vi "2ASK - 2PSK -2FSK.vi"() -> ()   [LabVIEW 2024]
uses:
  <vilib>/Analysis/NI_AALBase.lvlib
panel:
  in  "Stop":bool
  in  "nbre d'échantillons":i32=1000
  in  "Fréquence (f)":dbl=20.0
  in  "Amplitude (A)":dbl=4.0
  in  "Fréquence (f0)":dbl=20.0
  in  "Fréquence (f1)":dbl=60.0
  in  "nbre d'échantillons":i32=1000
  in  "Amplitude (A)":dbl=5.0
  out "Suite binaire (LED)":bool[](array[boolean]) caption="Array 4"
  in  "Fréquence (f)":dbl=40.0
  in  "nbre d'échantillons":i32=1000
  in  "Amplitude (A0)":dbl=2.0
  in  "Amplitude (A1)":dbl=8.0
  in  "Type de Modulation":u16(ring) items=["2-FSK", "2-PSK", "2-ASK"]
  out "Signal Résultant":dbl[](graph)
  out "Signal Porteur N°1":dbl[](graph)
  out "Inverse du signal binaire x Signal porteur N°2":dbl[](graph)
  out "Signal binaire":dbl[](graph)
  out "Signal Porteur N°2":dbl[](graph)
  out "Signal binaire x Signal porteur N°1":dbl[](graph)
  in  "Suite binaire":bool[](array[boolean])=[TRUE, TRUE, TRUE, FALSE, FALSE, FALSE, FALSE, TRUE, TRUE, TRUE]
  # "Paramètres des signaux porteurs"
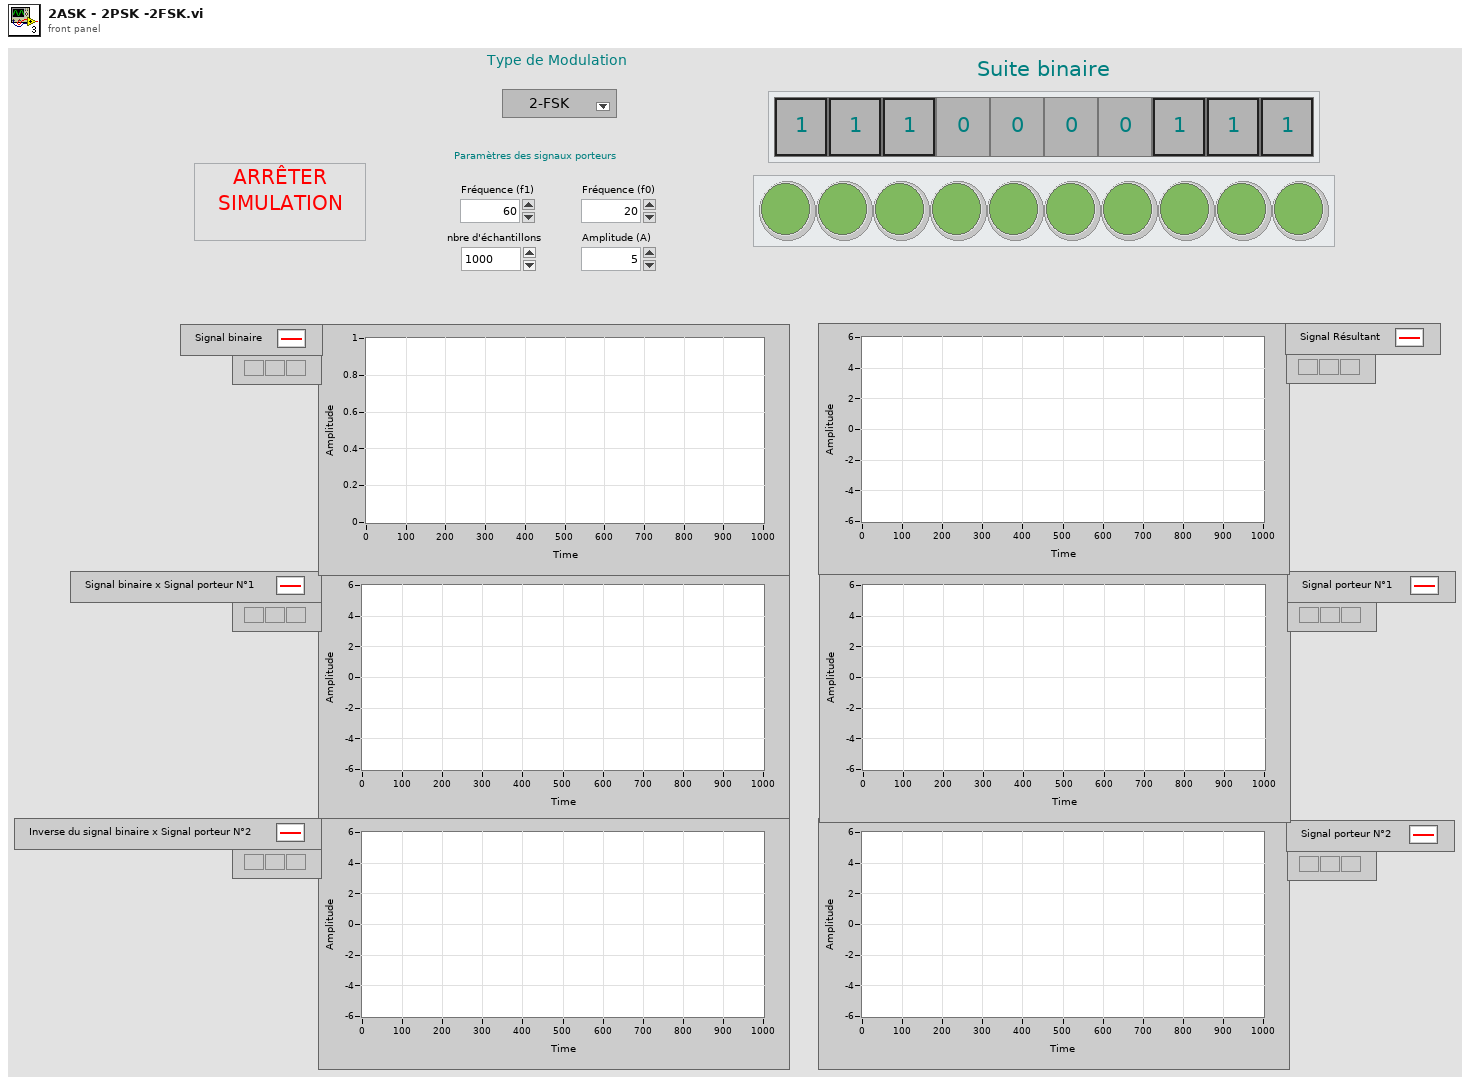
[diagram p1: front panel]
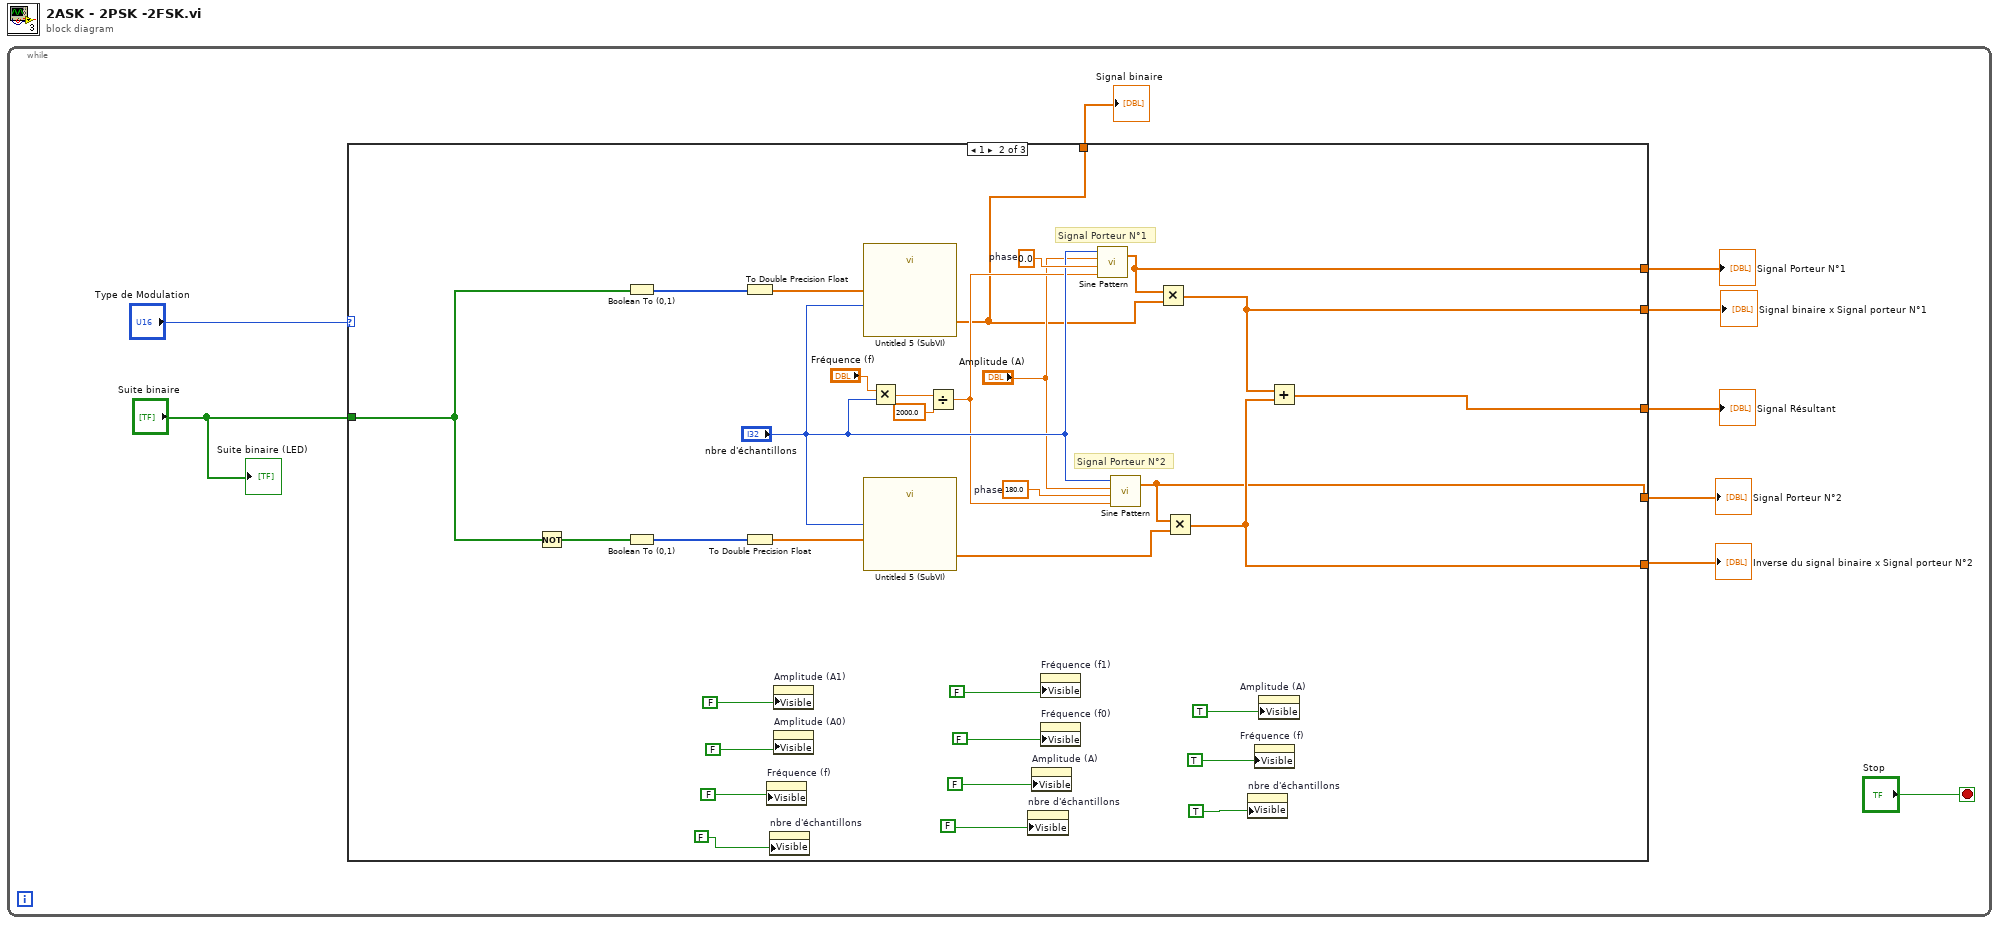
[diagram p0: block diagram]
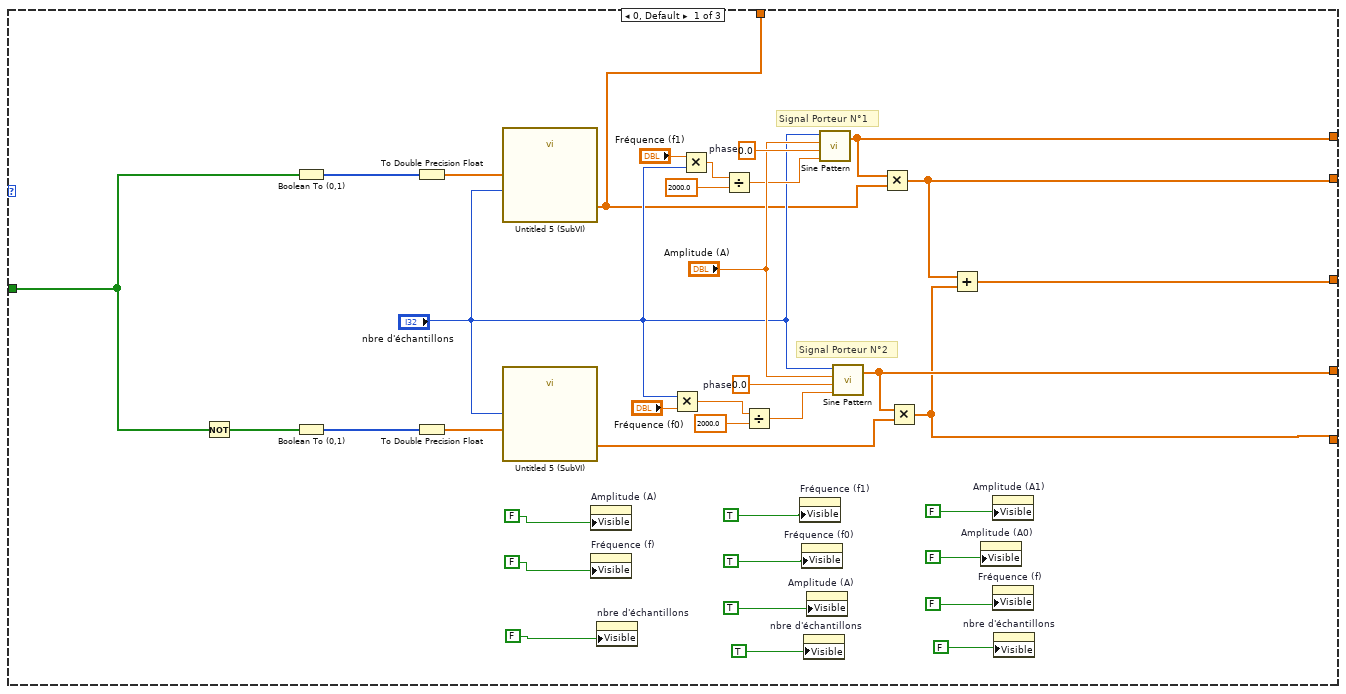
[diagram p2: hidden frame]
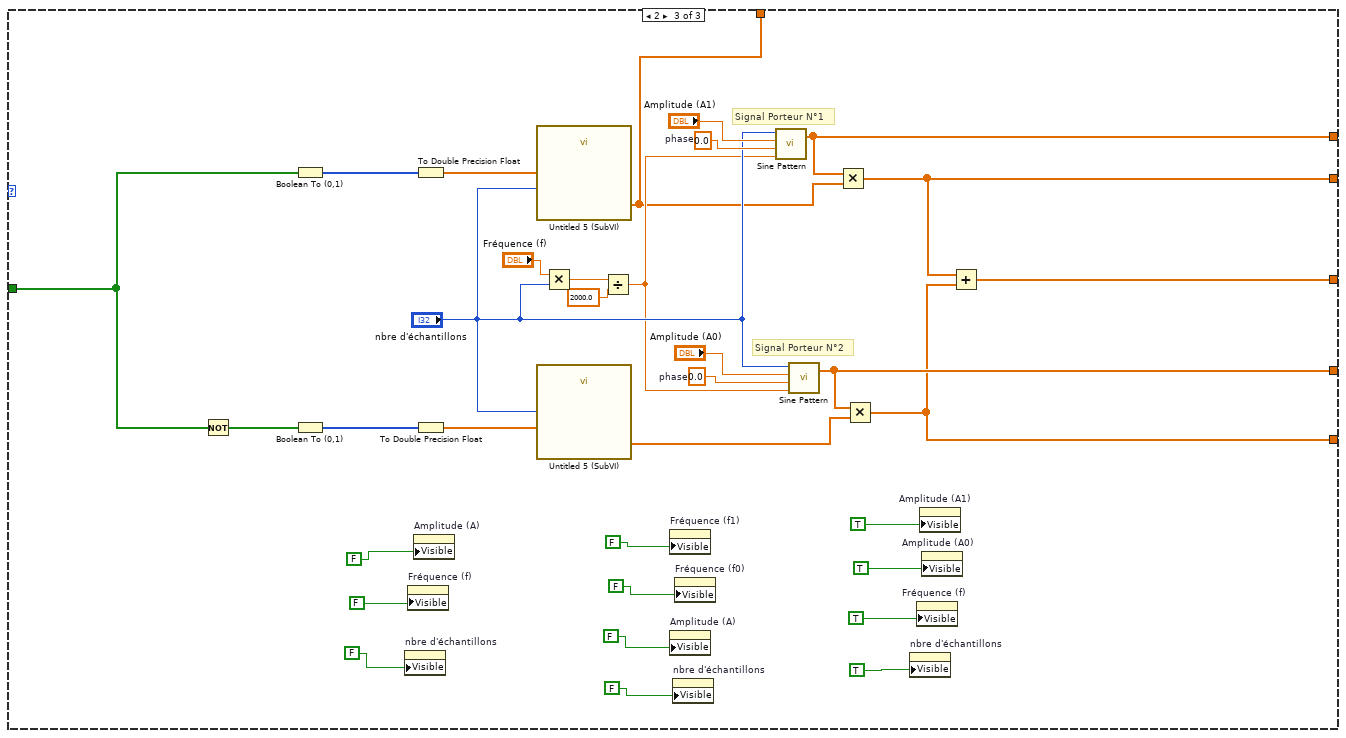
[diagram p3: hidden frame]
diagram:
  n1 = while {
    stop <- "Stop" stop-if-true
    n2 = case shown="1" "Type de Modulation" {
      tunnel: [w35 w46 w80] -> w1
      tunnel: [w36 w59 w83] -> w8
      tunnel: [w34 w60 w79] -> w5
      tunnel: [w33 w57 w81] -> w7
      tunnel: [w37 w58 w82] -> w6
      tunnel: "Suite binaire" -> [w38 w61 w92]
      tunnel: [w10 w47 w78] -> w2
      frame 0, Default {
        w40 = 0.0  # phase
        w32 = 0.0  # phase
        # "Signal Porteur N°1"
        # "Signal Porteur N°2"
        n3 = Not(x=w38) -> (.not. x?=w41:bool[])
        n4 = Boolean To (0,1)(Boolean=w38) -> (0, 1=w42:i16[])
        n5 = Boolean To (0,1)(Boolean=w41) -> (0, 1=w45:i16[])
        n6 = To Double Precision Float(number=w42) -> (double precision float=w43:dbl[])
        n7 = To Double Precision Float(number=w45) -> (double precision float=w44:dbl[])
        n8 = call "Untitled 5 (SubVI).vi"("Array in"=w43, "x"="nbre d'échantillons") -> ("Array out"=w10:dbl[])  [unwired: 9 in]
        n9 = call "Untitled 5 (SubVI).vi"("Array in"=w44, "x"="nbre d'échantillons") -> ("Array out"=w39:dbl[])  [unwired: 9 in]
        n10 = property on="Amplitude (A)" class="DigNum (strict)"("Visible"=FALSE) -> ()  [unwired: 2 in, 2 out]
        n11 = property on="Fréquence (f)" class="DigNum (strict)"("Visible"=FALSE) -> ()  [unwired: 2 in, 2 out]
        n12 = property on="nbre d'échantillons" class="DigNum (strict)"("Visible"=FALSE) -> ()  [unwired: 2 in, 2 out]
        n13 = Multiply(x="nbre d'échantillons", y="Fréquence (f0)") -> (x*y=w24:dbl)
        n14 = Multiply(x="Fréquence (f1)", y="nbre d'échantillons") -> (x*y=w26:dbl)
        n15 = Divide(x=w26, y=2000.0) -> (x/y=w30:dbl)
        n16 = Divide(x=w24, y=2000.0) -> (x/y=w29:dbl)
        n17 = property on="Fréquence (f1)" class="DigNum (strict)"("Visible"=TRUE) -> ()  [unwired: 2 in, 2 out]
        n18 = property on="Fréquence (f0)" class="DigNum (strict)"("Visible"=TRUE) -> ()  [unwired: 2 in, 2 out]
        n19 = property on="nbre d'échantillons" class="DigNum (strict)"("Visible"=TRUE) -> ()  [unwired: 2 in, 2 out]
        n20 = property on="Amplitude (A)" class="DigNum (strict)"("Visible"=TRUE) -> ()  [unwired: 2 in, 2 out]
        n21 = call <vilib>:"Sine Pattern.vi"("cycles"=w30, "phase(degrees)"=w40, "amplitude"="Amplitude (A)", "samples"="nbre d'échantillons") -> ("Sinusoidal Pattern"=w33:dbl[])  [unwired: 1 out]
        n22 = call <vilib>:"Sine Pattern.vi"("cycles"=w29, "phase(degrees)"=w32, "amplitude"="Amplitude (A)", "samples"="nbre d'échantillons") -> ("Sinusoidal Pattern"=w35:dbl[])  [unwired: 1 out]
        n23 = Multiply(x=w33, y=w10) -> (x*y=w37:dbl[])
        n24 = Multiply(x=w35, y=w39) -> (x*y=w34:dbl[])
        n25 = Add(x=w37, y=w34) -> (x+y=w36:dbl[])
        n26 = property on="Amplitude (A0)" class="DigNum (strict)"("Visible"=FALSE) -> ()  [unwired: 2 in, 2 out]
        n27 = property on="Amplitude (A1)" class="DigNum (strict)"("Visible"=FALSE) -> ()  [unwired: 2 in, 2 out]
        n28 = property on="Fréquence (f)" class="DigNum (strict)"("Visible"=FALSE) -> ()  [unwired: 2 in, 2 out]
        n29 = property on="nbre d'échantillons" class="DigNum (strict)"("Visible"=FALSE) -> ()  [unwired: 2 in, 2 out]
      }
      frame 1 {
        w72 = 0.0  # phase
        w73 = 180.0  # phase
        # "Signal Porteur N°1"
        # "Signal Porteur N°2"
        n30 = Not(x=w61) -> (.not. x?=w77:bool[])
        n31 = Boolean To (0,1)(Boolean=w61) -> (0, 1=w76:i16[])
        n32 = Boolean To (0,1)(Boolean=w77) -> (0, 1=w64:i16[])
        n33 = To Double Precision Float(number=w76) -> (double precision float=w75:dbl[])
        n34 = To Double Precision Float(number=w64) -> (double precision float=w74:dbl[])
        n35 = property on="Fréquence (f)" class="DigNum (strict)"("Visible"=FALSE) -> ()  [unwired: 2 in, 2 out]
        n36 = property on="nbre d'échantillons" class="DigNum (strict)"("Visible"=FALSE) -> ()  [unwired: 2 in, 2 out]
        n37 = property on="Amplitude (A1)" class="DigNum (strict)"("Visible"=FALSE) -> ()  [unwired: 2 in, 2 out]
        n38 = property on="Amplitude (A0)" class="DigNum (strict)"("Visible"=FALSE) -> ()  [unwired: 2 in, 2 out]
        n39 = call "Untitled 5 (SubVI).vi"("Array in"=w75, "x"="nbre d'échantillons") -> ("Array out"=w47:dbl[])  [unwired: 9 in]
        n40 = call "Untitled 5 (SubVI).vi"("Array in"=w74, "x"="nbre d'échantillons") -> ("Array out"=w62:dbl[])  [unwired: 9 in]
        n41 = Multiply(x="Fréquence (f)", y="nbre d'échantillons") -> (x*y=w69:dbl)
        n42 = Divide(x=w69, y=2000.0) -> (x/y=w67:dbl)
        n43 = property on="nbre d'échantillons" class="DigNum (strict)"("Visible"=FALSE) -> ()  [unwired: 2 in, 2 out]
        n44 = property on="Amplitude (A)" class="DigNum (strict)"("Visible"=FALSE) -> ()  [unwired: 2 in, 2 out]
        n45 = property on="Fréquence (f1)" class="DigNum (strict)"("Visible"=FALSE) -> ()  [unwired: 2 in, 2 out]
        n46 = property on="Fréquence (f0)" class="DigNum (strict)"("Visible"=FALSE) -> ()  [unwired: 2 in, 2 out]
        n47 = call <vilib>:"Sine Pattern.vi"("cycles"=w67, "phase(degrees)"=w72, "amplitude"="Amplitude (A)", "samples"="nbre d'échantillons") -> ("Sinusoidal Pattern"=w57:dbl[])  [unwired: 1 out]
        n48 = call <vilib>:"Sine Pattern.vi"("cycles"=w67, "phase(degrees)"=w73, "amplitude"="Amplitude (A)", "samples"="nbre d'échantillons") -> ("Sinusoidal Pattern"=w46:dbl[])  [unwired: 1 out]
        n49 = Multiply(x=w57, y=w47) -> (x*y=w58:dbl[])
        n50 = Multiply(x=w46, y=w62) -> (x*y=w60:dbl[])
        n51 = property on="nbre d'échantillons" class="DigNum (strict)"("Visible"=TRUE) -> ()  [unwired: 2 in, 2 out]
        n52 = property on="Fréquence (f)" class="DigNum (strict)"("Visible"=TRUE) -> ()  [unwired: 2 in, 2 out]
        n53 = property on="Amplitude (A)" class="DigNum (strict)"("Visible"=TRUE) -> ()  [unwired: 2 in, 2 out]
        n54 = Add(x=w58, y=w60) -> (x+y=w59:dbl[])
      }
      frame 2 {
        w102 = 0.0  # phase
        w104 = 0.0  # phase
        # "Signal Porteur N°1"
        # "Signal Porteur N°2"
        n55 = Not(x=w92) -> (.not. x?=w110:bool[])
        n56 = Boolean To (0,1)(Boolean=w92) -> (0, 1=w109:i16[])
        n57 = Boolean To (0,1)(Boolean=w110) -> (0, 1=w94:i16[])
        n58 = property on="nbre d'échantillons" class="DigNum (strict)"("Visible"=FALSE) -> ()  [unwired: 2 in, 2 out]
        n59 = property on="Fréquence (f)" class="DigNum (strict)"("Visible"=FALSE) -> ()  [unwired: 2 in, 2 out]
        n60 = property on="Amplitude (A)" class="DigNum (strict)"("Visible"=FALSE) -> ()  [unwired: 2 in, 2 out]
        n61 = To Double Precision Float(number=w109) -> (double precision float=w108:dbl[])
        n62 = To Double Precision Float(number=w94) -> (double precision float=w107:dbl[])
        n63 = call "Untitled 5 (SubVI).vi"("Array in"=w108, "x"="nbre d'échantillons") -> ("Array out"=w78:dbl[])  [unwired: 9 in]
        n64 = call "Untitled 5 (SubVI).vi"("Array in"=w107, "x"="nbre d'échantillons") -> ("Array out"=w93:dbl[])  [unwired: 9 in]
        n65 = Multiply(x="Fréquence (f)", y="nbre d'échantillons") -> (x*y=w99:dbl)
        n66 = Divide(x=w99, y=2000.0) -> (x/y=w97:dbl)
        n67 = property on="Fréquence (f1)" class="DigNum (strict)"("Visible"=FALSE) -> ()  [unwired: 2 in, 2 out]
        n68 = property on="Amplitude (A)" class="DigNum (strict)"("Visible"=FALSE) -> ()  [unwired: 2 in, 2 out]
        n69 = property on="nbre d'échantillons" class="DigNum (strict)"("Visible"=FALSE) -> ()  [unwired: 2 in, 2 out]
        n70 = property on="Fréquence (f0)" class="DigNum (strict)"("Visible"=FALSE) -> ()  [unwired: 2 in, 2 out]
        n71 = call <vilib>:"Sine Pattern.vi"("cycles"=w97, "phase(degrees)"=w102, "amplitude"="Amplitude (A1)", "samples"="nbre d'échantillons") -> ("Sinusoidal Pattern"=w81:dbl[])  [unwired: 1 out]
        n72 = call <vilib>:"Sine Pattern.vi"("cycles"=w97, "phase(degrees)"=w104, "amplitude"="Amplitude (A0)", "samples"="nbre d'échantillons") -> ("Sinusoidal Pattern"=w80:dbl[])  [unwired: 1 out]
        n73 = Multiply(x=w81, y=w78) -> (x*y=w82:dbl[])
        n74 = Multiply(x=w80, y=w93) -> (x*y=w79:dbl[])
        n75 = property on="nbre d'échantillons" class="DigNum (strict)"("Visible"=TRUE) -> ()  [unwired: 2 in, 2 out]
        n76 = property on="Fréquence (f)" class="DigNum (strict)"("Visible"=TRUE) -> ()  [unwired: 2 in, 2 out]
        n77 = property on="Amplitude (A1)" class="DigNum (strict)"("Visible"=TRUE) -> ()  [unwired: 2 in, 2 out]
        n78 = property on="Amplitude (A0)" class="DigNum (strict)"("Visible"=TRUE) -> ()  [unwired: 2 in, 2 out]
        n79 = Add(x=w82, y=w79) -> (x+y=w83:dbl[])
      }
    }
    "Signal binaire x Signal porteur N°1" <- w6
    "Signal Porteur N°1" <- w7
    "Signal Porteur N°2" <- w1
    "Signal Résultant" <- w8
    "Inverse du signal binaire x Signal porteur N°2" <- w5
    "Signal binaire" <- w2
    "Suite binaire (LED)" <- "Suite binaire"
  }
